vi "Front Initialize.vi"() -> (0 "Back Grabber Total":T1)   [LabVIEW 2010]
uses:
  <vilib>/NXT/Subs/MotorXNode.Servo Type.ctl
  <vilib>/NXT/Subs/MotorXNode.1Servo.ctl
  <vilib>/NXT/Subs/LVHSConnector.ctl
  <vilib>/NXT/NXTIO Xnodes/NXTIONodeSubVIs/TETRIX IO Move Servos.vi
  <vilib>/NXT/NXTIO Xnodes/NXTIOXNode/NXTIO.xnode
  <vilib>/NXT/NXTIO Xnodes/AddressXNode/NXTIOAddress.xnode
  4150_RingItUp_State/4150_RingItUp_State.lvrbt
  grabber positions.ctl
  Grabber Total.ctl
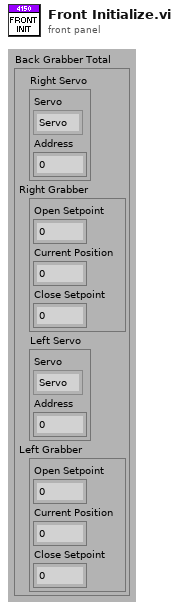
[diagram p1: front panel]
types:
  T1 = typedef "Grabber Total.ctl" = cluster{"Right Servo":cluster{"Servo":T2, "Address":i16}, "Right Grabber":T3, "Left Servo":cluster{"Servo":T2, "Address":i16}, "Left Grabber":T3}
  T2 = typedef "MotorXNode.Servo Type.ctl" = enum16{"Servo"}
  T3 = typedef "grabber positions.ctl" = cluster{"Open Setpoint":u8, "Current Position":u8, "Close Setpoint":u8}
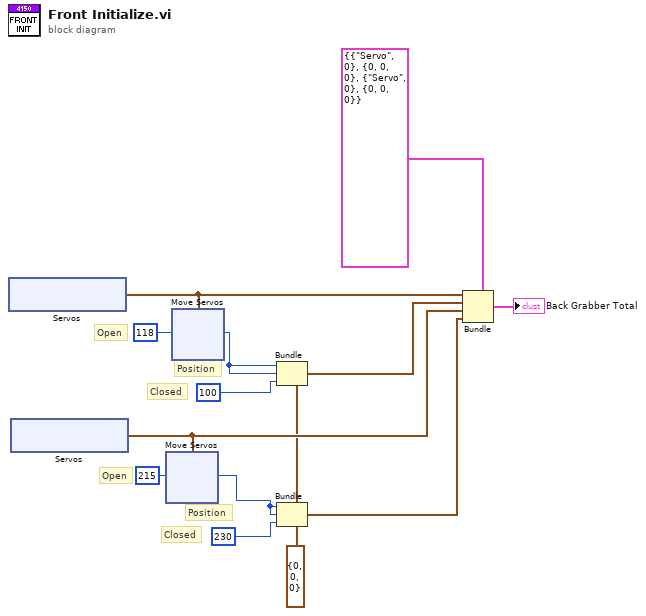
[diagram p0: block diagram]
diagram:
  w1 = T3 {"Open Setpoint"=0, "Current Position"=0, "Close Setpoint"=0} ("Left Grabber")
  w3 = u8 215 ("Position 1")
  w6 = u8 118 ("Position 1")
  # "Open"
  # "Closed"
  # "Position"
  # "Closed"
  # "Position"
  # "Open"
  n1 = xnode "Servos"() -> ("Servo"=w7:cluster{"Servo":T2, "Address":i16})
  n2 = xnode "Servos"() -> ("Servo"=w9:cluster{"Servo":T2, "Address":i16})
  n3 = xnode ("Move Servos")("Position 1"=w3, "Servos"=w9) -> ()  [unwired: 1 in, 1 out]
  n4 = xnode ("Move Servos")("Position 1"=w6, "Servos"=w7) -> ()  [unwired: 1 in, 1 out]
  n5 = Bundle(cluster=w1, "Open Setpoint"=w6, "Current Position"=w6, "Close Setpoint"=u8 100 ("Position 1")) -> (w8:T3)
  n6 = Bundle(cluster=w1, "Open Setpoint"=w3, "Current Position"=w3, "Close Setpoint"=u8 230 ("Position 1")) -> (w10:T3)
  n7 = Bundle(cluster=T1 {"Right Servo"={"Servo"=enum."Servo", "Address"=0}, "Right Grabber"={"Open Setpoint"=0, "Current Position"=0, "Close Setpoint"=0}, "Left Servo"={"Servo"=enum."Servo", "Address"=0}, "Left Grabber"={"Open Setpoint"=0, "Current Position"=0, "Close Setpoint"=0}}, "Right Servo"=w7, "Right Grabber"=w8, "Left Servo"=w9, "Left Grabber"=w10) -> (→"Back Grabber Total":T1)
